vi "Actor Core.vi"(8 "error in":errorcluster, 11 "Signal Analysis in":refnum<class "Signal Analysis.lvclass">) -> (0 "error out":errorcluster, 3 "Actor out":refnum<class "Actor.lvclass">)   [LabVIEW 2023, in "Data Analysis.lvlib" / "Signal Analysis.lvlib" / "Signal Analysis.lvclass"]
doc: "(<B>Filename</B>: Actor Framework.lvlib:Actor.lvclass:Actor Core.vi)\n\nReceives messages to the actor, reacts to them, and initiates any error handling that may shut the actor down.\n\nDescendant classes may override this VI to append parallel tasks for the actor to complete while it handles messages. Overrides use the Call Parent Class Method node."
uses:
  Signal Analysis.lvclass
  C:/Program Files/National Instruments/LabVIEW 2023/vi.lib/ActorFramework/Actor/Actor.lvclass
  <vilib>/ActorFramework/Actor/Actor.lvclass
  Signal Analysis.lvclass/Signal Analysis.ctl
  <vilib>/ActorFramework/Actor/Actor.lvclass/Actor.ctl
  <vilib>/ActorFramework/Message Enqueuer/Message Enqueuer.lvclass/Message Enqueuer.ctl
  Subpanel-Abstract Messages/Insert SP Msg/Insert SP Msg.lvclass/Insert SP Msg.ctl
  Signal Analysis Messages/Schema Update Msg/Schema Update Msg.lvclass/Schema Update Msg.ctl
  Signal Analysis Messages/Plot Signal Msg/Plot Signal Msg.lvclass/Plot Signal Msg.ctl
  <vilib>/ActorFramework/Message Enqueuer/Init from Existing Queue.vi
  <vilib>/ActorFramework/Message Enqueuer/Enqueue.vi
  Subpanel-Abstract Messages/Insert SP Msg/Insert SP Msg.lvclass
  C:/Program Files/National Instruments/LabVIEW 2023/vi.lib/ActorFramework/Message/Message.lvclass
  Signal Analysis Messages/Schema Update Msg/Schema Update Msg.lvclass
  Signal Analysis Messages/Plot Signal Msg/Plot Signal Msg.lvclass
  <vilib>/ActorFramework/Message Priority Queue/Priority Enqueue.vi
  <vilib>/ActorFramework/Message Enqueuer/Message Enqueuer.lvclass
  Subpanel-Abstract/Subpanel-Abstract.lvclass
panel:
  in  "Select All Socket button":bool=TRUE caption="Checkbox"
  in  "Visible Plots":T1={"Socket 0"=TRUE, "Socket 1"=TRUE, "Socket 2"=TRUE, "Socket 3"=TRUE, "Socket 4"=TRUE, "Socket 5"=TRUE}
  out "XY Graph 2":cluster{dbl[], dbl[]}[](graph) caption="XY Graph - Dark"
  in  "Plot Signal 2":bool
  in  "Signal Name 2":string(combo)
  out "XY Graph":cluster{dbl[], dbl[]}[](graph) caption="XY Graph - Dark"
  in  "Plot Signal":bool
  in  "Signal Name":string(combo)
  in  "Stop":bool
  # "Signal Analysis"
  # "*Frame Type and Test Mode filters are Mantatory."
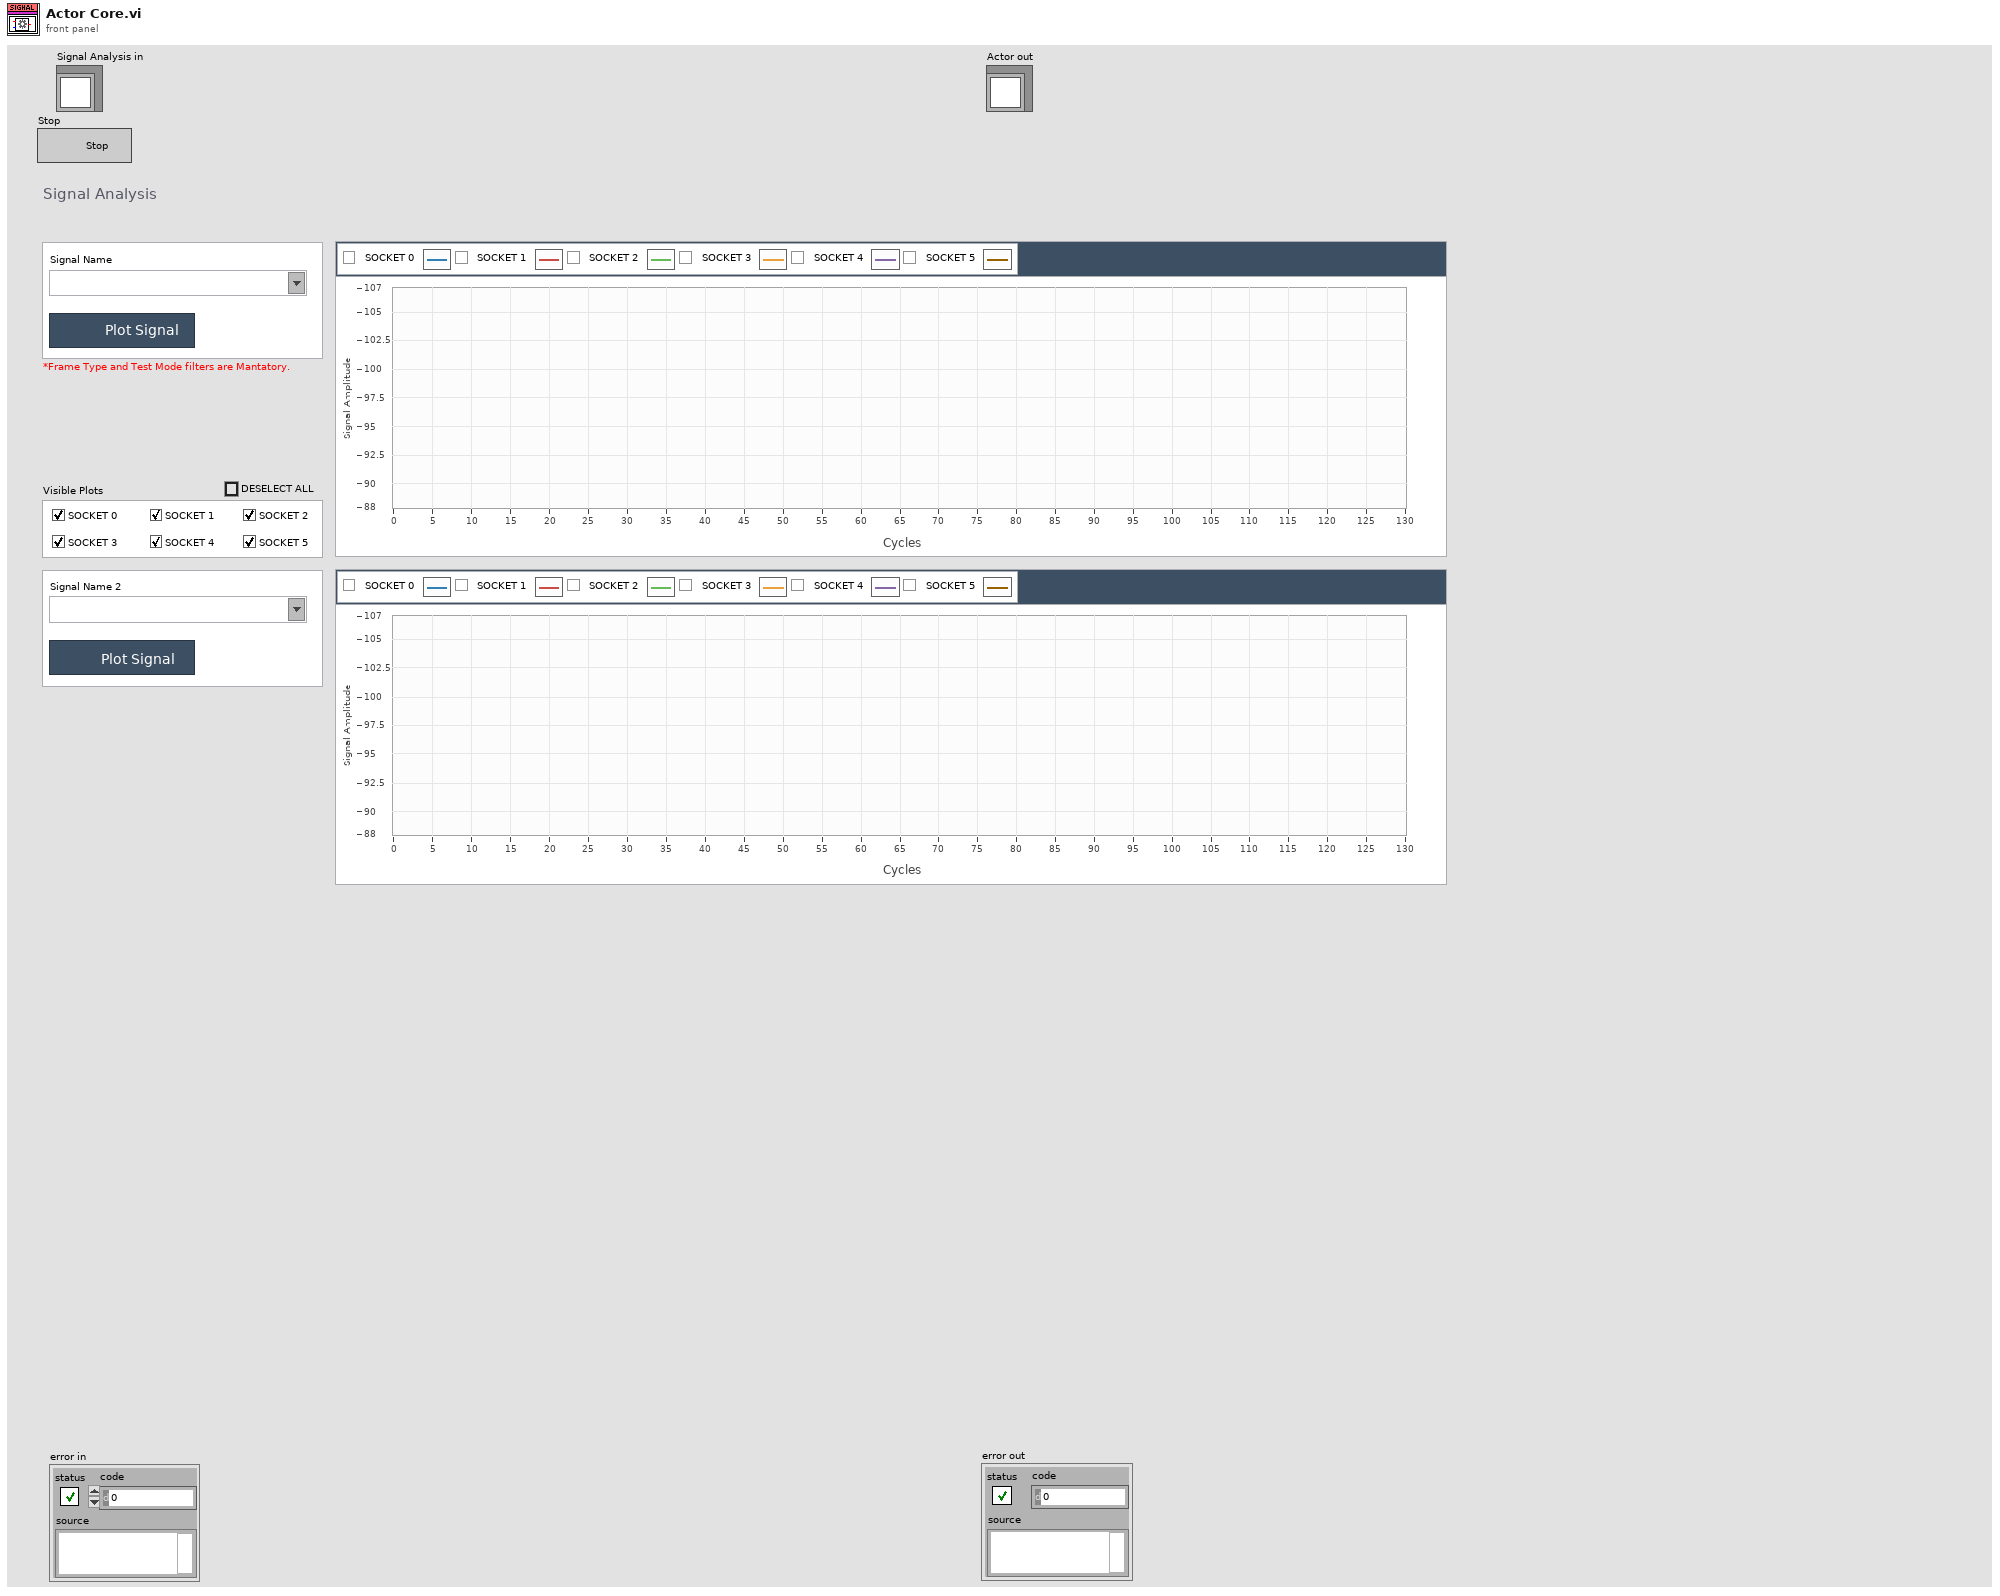
[diagram p1: front panel]
types:
  T1 = cluster{"Socket 0":bool, "Socket 1":bool, "Socket 2":bool, "Socket 3":bool, "Socket 4":bool, "Socket 5":bool}
  T2 = enum8{"Enabled", "Disabled", "Disabled and Grayed Out"}
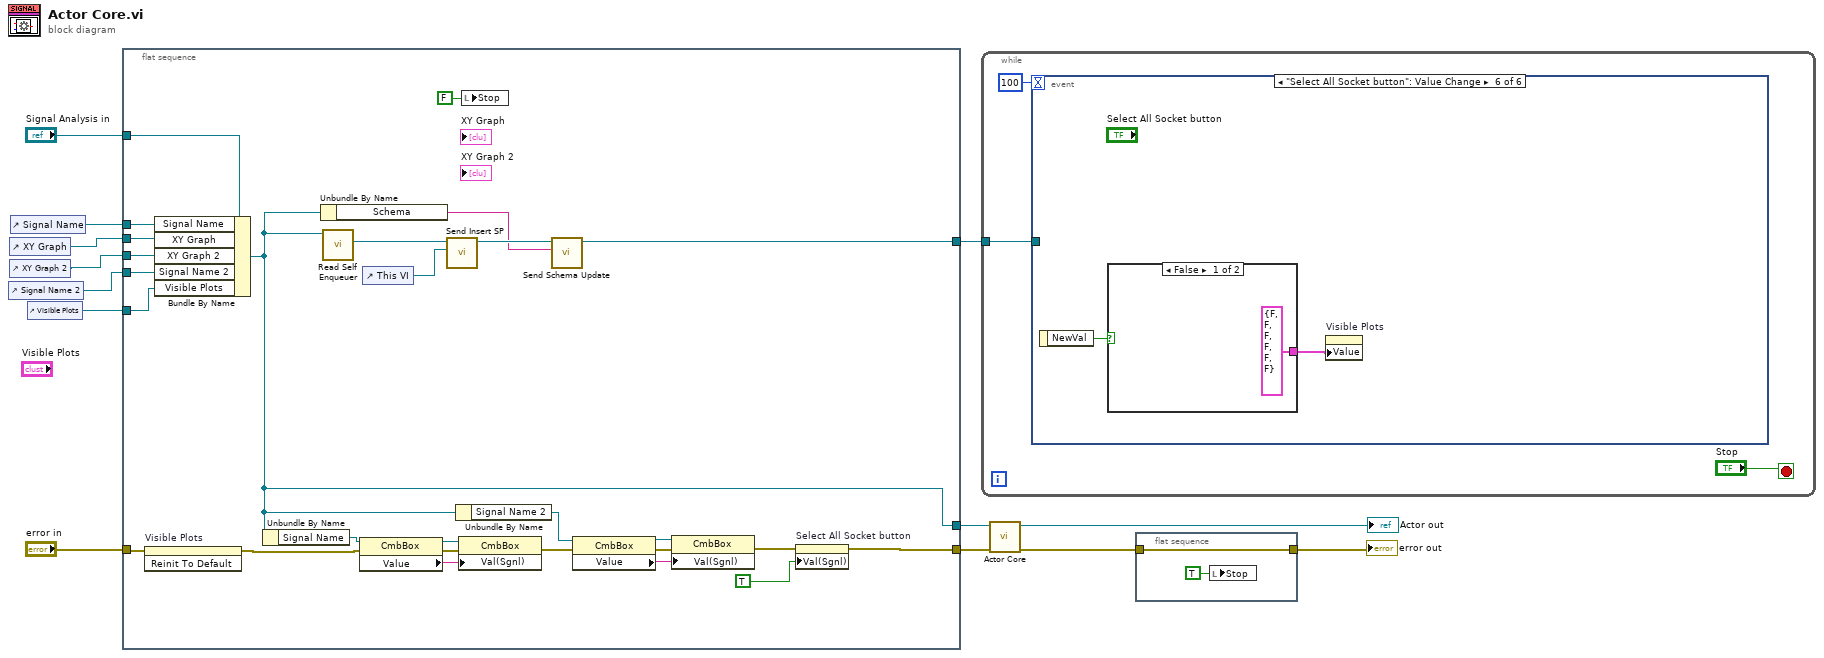
[diagram p0: block diagram]
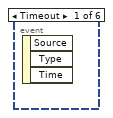
[diagram p2: hidden frame]
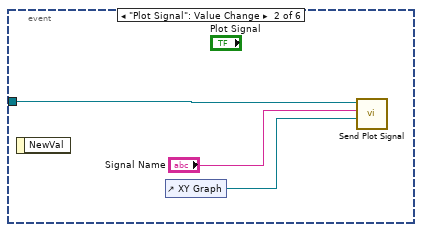
[diagram p3: hidden frame]
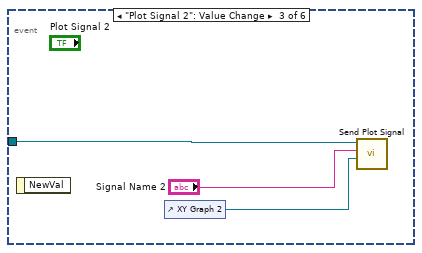
[diagram p4: hidden frame]
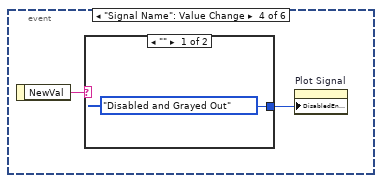
[diagram p5: hidden frame]
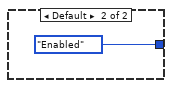
[diagram p6: hidden frame]
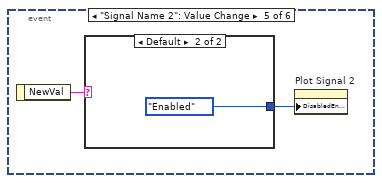
[diagram p7: hidden frame]
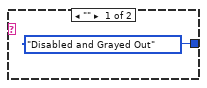
[diagram p8: hidden frame]
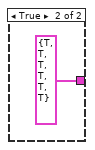
[diagram p9: hidden frame]
diagram:
  n1 = control-ref of="Signal Name 2"() -> (w3:refnum<vi>)
  n2 = control-ref of="XY Graph"() -> (w4:refnum<vi>)
  n3 = control-ref of="XY Graph 2"() -> (w2:refnum<vi>)
  n4 = control-ref of="Signal Name"() -> (w5:refnum<vi>)
  n5 = control-ref of="Visible Plots"() -> (w1:refnum<vi>)
  n6 = flat-sequence {
    tunnel: "error in" -> [w17]
    tunnel: [w15] -> w11
    tunnel: "Signal Analysis in" -> [w37]
    tunnel: [w23] -> w9
    tunnel: [w33] -> w6
    tunnel: w5 -> [w36]
    tunnel: w4 -> [w35]
    tunnel: w2 -> [w31]
    tunnel: w3 -> [w30]
    tunnel: w1 -> [w19]
    frame #0 {
      n7 = invoke on="Visible Plots" class="Clust (strict)" method="Reinit To Default"(error in=w17) -> (error out=w18:errorcluster)  [unwired: 2 in, 2 out]
      n8 = Bundle By Name(cluster=w37, "Signal Name"=w36, "XY Graph"=w35, "XY Graph 2"=w31, "Signal Name 2"=w30, "Visible Plots"=w19) -> (w23:refnum<class "Signal Analysis.lvclass">)
      n9 = Unbundle By Name(w23) -> ("Signal Name"=w29:refnum<vi>)
      n10 = Unbundle By Name(w23) -> ("Schema"=w32:string)
      n11 = call <vilib>:"Read Self Enqueuer.vi"("Actor"=w23) -> ("Self Enqueuer"=w39:refnum<class "Message Enqueuer.lvclass">)  [unwired: 10 in]
      n12 = property class="CmbBox"(reference=w29, error in=w18) -> (reference out=w28:refnum<vi>, error out=w27:errorcluster, "Value"=w26:string)
      n13 = control-ref of="This VI"() -> (w38:refnum<vi>)
      n14 = call "Send Insert SP.vi"("VI Ref"=w38, "Message Enqueuer"=w39) -> ("Message Enqueuer out"=w34:refnum<class "Message Enqueuer.lvclass">)  [unwired: 8 in, 1 out]
      n15 = Unbundle By Name(w23) -> ("Signal Name 2"=w22:refnum<vi>)
      n16 = property class="CmbBox"(reference=w28, error in=w27, "Val(Sgnl)"=w26) -> (error out=w21:errorcluster)  [unwired: 1 out]
      n17 = local write "Stop"(FALSE ("Stop")) -> ()
      n18 = call "Send Schema Update.vi"("Schema"=w32, "Message Enqueuer"=w34) -> ("Message Enqueuer out"=w33:refnum<class "Message Enqueuer.lvclass">)  [unwired: 8 in, 1 out]
      n19 = property class="CmbBox"(reference=w22, error in=w21) -> (reference out=w20:refnum<vi>, error out=w24:errorcluster, "Value"=w25:string)
      n20 = property class="CmbBox"(reference=w20, error in=w24, "Val(Sgnl)"=w25) -> (error out=w16:errorcluster)  [unwired: 1 out]
      n21 = property on="Select All Socket button" class="Bool (strict)"(error in=w16, "Val(Sgnl)"=TRUE ("Value (Signaling)")) -> (error out=w15:errorcluster)  [unwired: 1 in, 1 out]
    }
  }
  n22 = while {
    tunnel: w6 -> [w41]
    stop <- "Stop" stop-if-true
    n23 = event shown="[5] \"Select All Socket button\": Value Change" {
      selector: _ -> [_ _ _ _ _ _]
      dyn-events: _ -> [_ _ _ _ _ _]
      timeout: 100 -> [_ _ _ _ _ _]
      tunnel: w41 -> [_ w46 w49 _ _ _]
      event Timeout {
        n24 = event-data() -> ()  [unwired: 1 in, 3 out]
      }
      event "Plot Signal": Value Change {
        n25 = event-data() -> ()  [unwired: 1 in, 1 out]
        n26 = control-ref of="XY Graph"() -> (w44:refnum<vi>)
        n27 = call "Send Plot Signal.vi"("XY Graph"=w44, "Signal Name"="Signal Name", "Message Enqueuer"=w46) -> ()  [unwired: 7 in, 2 out]
      }
      event "Plot Signal 2": Value Change {
        n28 = event-data() -> ()  [unwired: 1 in, 1 out]
        n29 = control-ref of="XY Graph 2"() -> (w47:refnum<vi>)
        n30 = call "Send Plot Signal.vi"("XY Graph"=w47, "Signal Name"="Signal Name 2", "Message Enqueuer"=w49) -> ()  [unwired: 7 in, 2 out]
      }
      event "Signal Name": Value Change {
        n31 = event-data() -> ("NewVal"=w50:string)  [unwired: 1 in]
        n32 = case shown="\"\"" w50 {
          tunnel: [T2."Disabled and Grayed Out" ("Disabled") T2."Enabled" ("Disabled")] -> w51
          frame "" {
          }
          frame Default {
          }
        }
        n33 = property on="Plot Signal" class="Bool"("DisabledEnum"=w51) -> ()  [unwired: 2 in, 2 out]
      }
      event "Signal Name 2": Value Change {
        n34 = event-data() -> ("NewVal"=w54:string)  [unwired: 1 in]
        n35 = case shown="Default" w54 {
          tunnel: [T2."Disabled and Grayed Out" ("Disabled") T2."Enabled" ("Disabled")] -> w55
          frame "" {
          }
          frame Default {
          }
        }
        n36 = property on="Plot Signal 2" class="Bool"("DisabledEnum"=w55) -> ()  [unwired: 2 in, 2 out]
      }
      event "Select All Socket button": Value Change {
        n37 = event-data() -> ("NewVal"=w59:bool)  [unwired: 1 in]
        n38 = case shown="False" w59 {
          tunnel: [T1 {"Socket 0"=FALSE, "Socket 1"=FALSE, "Socket 2"=FALSE, "Socket 3"=FALSE, "Socket 4"=FALSE, "Socket 5"=FALSE} ("Visible Plots") T1 {"Socket 0"=TRUE, "Socket 1"=TRUE, "Socket 2"=TRUE, "Socket 3"=TRUE, "Socket 4"=TRUE, "Socket 5"=TRUE} ("Visible Plots")] -> w58
          frame False {
          }
          frame True {
          }
        }
        n39 = property on="Visible Plots" class="Clust (strict)"("Value"=w58) -> ()  [unwired: 2 in, 2 out]
      }
    }
  }
  n40 = call-parent "Actor Core.vi"("error in"=w11, "Actor in"=w9) -> ("error out"=w8:errorcluster, "Actor out"=→"Actor out":refnum<class "Actor.lvclass">)  [unwired: 8 in]
  n41 = flat-sequence {
    tunnel: w8 -> [w63]
    tunnel: [w63] -> w7
    frame #0 {
      n42 = local write "Stop"(TRUE ("Stop")) -> ()
    }
  }
  "error out" <- w7
